vi "To Upper & Lower Case part 6.vi"() -> ()   [LabVIEW 2020]
panel:
  out "all upper case string":string
  in  "string":string
  # "Part 6"
  # "To Upper & Lower Case"
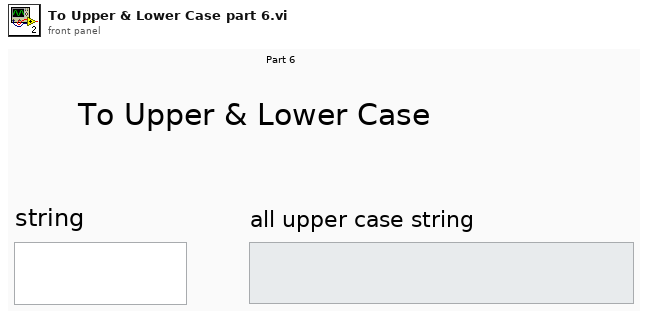
[diagram p1: front panel]
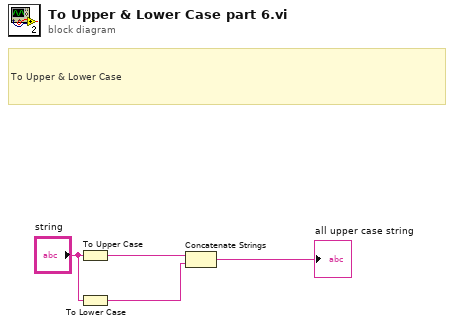
[diagram p0: block diagram]
diagram:
  # "To Upper & Lower Case"
  n1 = To Upper Case(1:"string") -> (0:w4:string)
  n2 = To Lower Case(string="string") -> (all lower case string=w3:string)
  n3 = Concatenate Strings "Concatenate Strings"(w4, w3) -> (→"all upper case string":string)
